vi "test.vi"() -> ()   [LabVIEW 2019]
panel:
  out "时间标识":timestamp
  out "错误输出":errorcluster
  out "VISA资源名称输出":refnum<visa-resource-name>
  in  "错误输入":errorcluster
  in  "VISA资源名称":refnum<visa-resource-name>
  in  "缓冲区名称":string(combo)
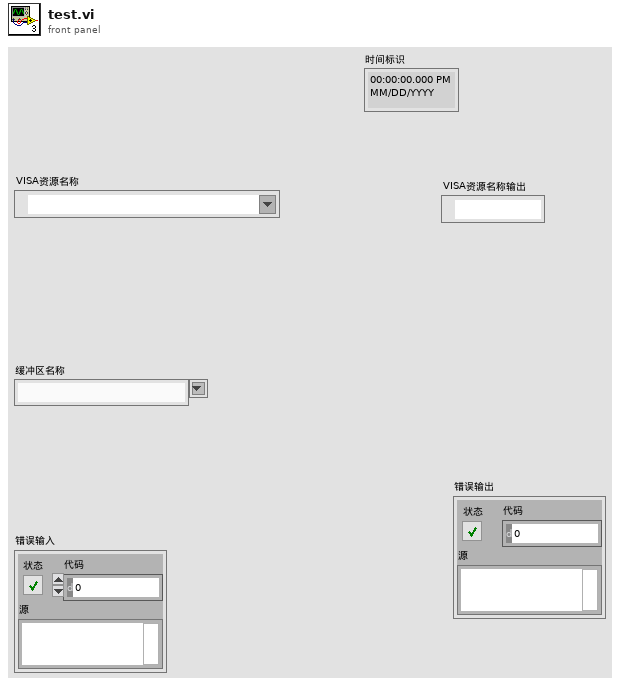
[diagram p1: front panel]
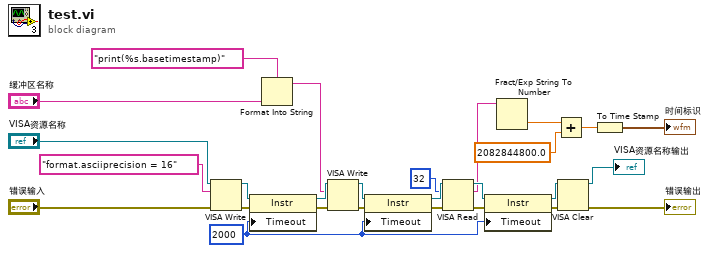
[diagram p0: block diagram]
diagram:
  w14 = u32 2000 ("General Settings:Timeout Value")
  n1 = VISA Write(VISA resource name="VISA资源名称", write buffer="format.asciiprecision = 16" ("格式字符串"), error in (no error)="错误输入") -> (VISA resource name out=w27:refnum<visa-resource-name>, error out=w26:errorcluster)  [unwired: 1 out]
  n2 = property class="Instr"(reference=w27, error in=w26, "Timeout"=w14) -> (reference out=w13:refnum<visa-resource-name>, error out=w12:errorcluster)
  n3 = Format Into String(format string="print(%s.basetimestamp)" ("格式字符串"), "缓冲区名称") -> (resulting string=w5:string)  [unwired: 2 in, 1 out]
  n4 = VISA Write(VISA resource name=w13, write buffer=w5, error in (no error)=w12) -> (VISA resource name out=w25:refnum<visa-resource-name>, error out=w24:errorcluster)  [unwired: 1 out]
  n5 = property class="Instr"(reference=w25, error in=w24, "Timeout"=w14) -> (reference out=w22:refnum<visa-resource-name>, error out=w23:errorcluster)
  n6 = VISA Read(VISA resource name=w22, byte count=u32 32 ("字节总数"), error in (no error)=w23) -> (VISA resource name out=w21:refnum<visa-resource-name>, read buffer=w8:string, error out=w20:errorcluster)  [unwired: 1 out]
  n7 = property class="Instr"(reference=w21, error in=w20, "Timeout"=w14) -> (reference out=w19:refnum<visa-resource-name>, error out=w18:errorcluster)
  n8 = Fract/Exp String To Number(string=w8) -> (number=w6:dbl)  [unwired: 3 in, 1 out]
  n9 = Add(x=w6, y=2082844800.0 ("x-y")) -> (x+y=w2:dbl)
  n10 = VISA Clear(VISA resource name=w19, error in (no error)=w18) -> (VISA resource name out=→"VISA资源名称输出":refnum<visa-resource-name>, error out=→"错误输出":errorcluster)
  n11 = To Time Stamp(1:w2) -> (0:→"时间标识":timestamp)
